vi "Lab Panel V5.28.vi"() -> ()   [LabVIEW 2013] (continued)
                          frame False {
                          }
                          frame True {
                            n3233 = Multiply(x=w5908, y=w5907) -> (x*y=w5906:dbl)
                            n3234 = Multiply(x=w5908, y=w5910) -> (x*y=w5909:dbl)
                          }
                        }
                        n3235 = case shown="True" w5876 {
                          tunnel: w5884 -> [w5912 w5917]
                          tunnel: w5885 -> [_ w5915]
                          tunnel: [w5912 w5916] -> w5882
                          tunnel: w5883 -> [w5911 w5914]
                          tunnel: [w5911 w5913] -> w5881
                          frame False {
                          }
                          frame True {
                            n3236 = Multiply(x=w5915, y=w5914) -> (x*y=w5913:dbl)
                            n3237 = Multiply(x=w5915, y=w5917) -> (x*y=w5916:dbl)
                          }
                        }
                        n3238 = local read "SIG LAB03-2"() -> (w5900:T2)
                        n3239 = local read "SIG LAB03-1"() -> (w5902:T2)
                        n3240 = Bundle By Name(cluster=w5902, "Tmp Live"=w5882, "Tmp Neut"=w5881) -> (w5901:T2)
                        n3241 = Bundle By Name(cluster=w5900, "Tmp Live"=w5878, "Tmp Neut"=w5877) -> (w5899:T2)
                        n3242 = local write "SIG LAB03-1"(w5901) -> ()
                        n3243 = local write "SIG LAB03-2"(w5899) -> ()
                      }
                      frame #4 {
                        n3244 = case shown="False" w5932 {
                          tunnel: [w5963 w5964] -> w5948
                          tunnel: w5931 -> [_ w5964]
                          frame False {
                            n3245 = local read "CAL LAB04"() -> (w5963:T14)
                          }
                          frame True {
                          }
                        }
                        n3246 = local read "LAB04 TEMP"() -> (w5938:T12)
                        n3247 = local read "TEMP LA04"() -> (w5939:T9)
                        n3248 = call "sub vi - temperature delay v4.vi"("2-run"=w5920, "1-run"=w5921, "temp values IN"=w5939, "temp signals"=w5938) -> ("T2-N"=w5933:dbl, "T2-L"=w5934:dbl, "T1-N"=w5935:dbl, "T1-L"=w5936:dbl, "temp values OUT"=w5937:T44)  [unwired: 3 in]
                        n3249 = Unbundle By Name(w5948) -> ("1 (TL) cal"=w5943:dbl, "1 (TN) cal"=w5942:dbl, "2 (TL) cal"=w5941:dbl, "2 (TN) cal"=w5940:dbl)  [unwired: 6 out]
                        n3250 = local write "TEMP LA04"(w5937) -> ()
                        n3251 = Multiply(x=w5936, y=w5943) -> (x*y=w5929:dbl)
                        n3252 = Multiply(x=w5935, y=w5942) -> (x*y=w5928:dbl)
                        n3253 = Multiply(x=w5934, y=w5941) -> (x*y=w5925:dbl)
                        n3254 = Multiply(x=w5933, y=w5940) -> (x*y=w5924:dbl)
                        n3255 = case shown="True" w5920 {
                          tunnel: w5925 -> [w5950 w5955]
                          tunnel: w5930 -> [_ w5953]
                          tunnel: [w5950 w5954] -> w5923
                          tunnel: w5924 -> [w5949 w5952]
                          tunnel: [w5949 w5951] -> w5922
                          frame False {
                          }
                          frame True {
                            n3256 = Multiply(x=w5953, y=w5952) -> (x*y=w5951:dbl)
                            n3257 = Multiply(x=w5953, y=w5955) -> (x*y=w5954:dbl)
                          }
                        }
                        n3258 = case shown="True" w5921 {
                          tunnel: w5929 -> [w5957 w5962]
                          tunnel: w5930 -> [_ w5960]
                          tunnel: [w5957 w5961] -> w5927
                          tunnel: w5928 -> [w5956 w5959]
                          tunnel: [w5956 w5958] -> w5926
                          frame False {
                          }
                          frame True {
                            n3259 = Multiply(x=w5960, y=w5959) -> (x*y=w5958:dbl)
                            n3260 = Multiply(x=w5960, y=w5962) -> (x*y=w5961:dbl)
                          }
                        }
                        n3261 = local read "SIG LAB04-2"() -> (w5945:T2)
                        n3262 = local read "SIG LAB04-1"() -> (w5947:T2)
                        n3263 = Bundle By Name(cluster=w5947, "Tmp Live"=w5927, "Tmp Neut"=w5926) -> (w5946:T2)
                        n3264 = Bundle By Name(cluster=w5945, "Tmp Live"=w5923, "Tmp Neut"=w5922) -> (w5944:T2)
                        n3265 = local write "SIG LAB04-1"(w5946) -> ()
                        n3266 = local write "SIG LAB04-2"(w5944) -> ()
                      }
                      frame #5 {
                        n3267 = case shown="False" w5977 {
                          tunnel: [w6008 w6009] -> w5993
                          tunnel: w5976 -> [_ w6009]
                          frame False {
                            n3268 = local read "CAL LAB05"() -> (w6008:T14)
                          }
                          frame True {
                          }
                        }
                        n3269 = local read "LAB05 TEMP"() -> (w5983:T12)
                        n3270 = local read "TEMP LA05"() -> (w5984:T9)
                        n3271 = call "sub vi - temperature delay v4.vi"("2-run"=w5965, "1-run"=w5966, "temp values IN"=w5984, "temp signals"=w5983) -> ("T2-N"=w5979:dbl, "T2-L"=w5980:dbl, "T1-N"=w5981:dbl, "T1-L"=w5982:dbl, "temp values OUT"=w5978:T44)  [unwired: 3 in]
                        n3272 = local write "TEMP LA05"(w5978) -> ()
                        n3273 = Unbundle By Name(w5993) -> ("1 (TL) cal"=w5985:dbl, "1 (TN) cal"=w5988:dbl, "2 (TL) cal"=w5987:dbl, "2 (TN) cal"=w5986:dbl)  [unwired: 6 out]
                        n3274 = Multiply(x=w5982, y=w5985) -> (x*y=w5974:dbl)
                        n3275 = Multiply(x=w5981, y=w5988) -> (x*y=w5973:dbl)
                        n3276 = Multiply(x=w5980, y=w5987) -> (x*y=w5970:dbl)
                        n3277 = Multiply(x=w5979, y=w5986) -> (x*y=w5969:dbl)
                        n3278 = case shown="True" w5965 {
                          tunnel: w5970 -> [w5995 w6000]
                          tunnel: w5975 -> [_ w5998]
                          tunnel: [w5995 w5999] -> w5968
                          tunnel: w5969 -> [w5994 w5997]
                          tunnel: [w5994 w5996] -> w5967
                          frame False {
                          }
                          frame True {
                            n3279 = Multiply(x=w5998, y=w5997) -> (x*y=w5996:dbl)
                            n3280 = Multiply(x=w5998, y=w6000) -> (x*y=w5999:dbl)
                          }
                        }
                        n3281 = case shown="True" w5966 {
                          tunnel: w5974 -> [w6002 w6007]
                          tunnel: w5975 -> [_ w6005]
                          tunnel: [w6002 w6006] -> w5972
                          tunnel: w5973 -> [w6001 w6004]
                          tunnel: [w6001 w6003] -> w5971
                          frame False {
                          }
                          frame True {
                            n3282 = Multiply(x=w6005, y=w6004) -> (x*y=w6003:dbl)
                            n3283 = Multiply(x=w6005, y=w6007) -> (x*y=w6006:dbl)
                          }
                        }
                        n3284 = local read "SIG LAB05-1"() -> (w5992:T2)
                        n3285 = Bundle By Name(cluster=w5992, "Tmp Live"=w5972, "Tmp Neut"=w5971) -> (w5991:T2)
                        n3286 = local read "SIG LAB05-2"() -> (w5990:T2)
                        n3287 = Bundle By Name(cluster=w5990, "Tmp Live"=w5968, "Tmp Neut"=w5967) -> (w5989:T2)
                        n3288 = local write "SIG LAB05-1"(w5991) -> ()
                        n3289 = local write "SIG LAB05-2"(w5989) -> ()
                      }
                      frame #6 {
                        w6110 = 150.0
                        # "check for thermocouple error, output >150 deg??"
                        n3290 = local read "SIG LAB01-2"() -> (w6119:T2)
                        n3291 = local read "SIG LAB04-1"() -> (w6113:T2)
                        n3292 = local read "SIG LAB04-2"() -> (w6114:T2)
                        n3293 = local read "SIG LAB01-1"() -> (w6120:T2)
                        n3294 = Unbundle(w6114) -> ("Tmp Live"=w6024:dbl, "Tmp Neut"=w6023:dbl)  [unwired: 3 out]
                        n3295 = Unbundle(w6119) -> ("Tmp Live"=w6045:dbl, "Tmp Neut"=w6043:dbl)  [unwired: 3 out]
                        n3296 = Unbundle(w6113) -> ("Tmp Live"=w6025:dbl, "Tmp Neut"=w6018:dbl)  [unwired: 3 out]
                        n3297 = Unbundle(w6120) -> ("Tmp Live"=w6048:dbl, "Tmp Neut"=w6046:dbl)  [unwired: 3 out]
                        n3298 = Absolute Value(x=w6025) -> (abs(x)=w6019:dbl)
                        n3299 = Absolute Value(x=w6018) -> (abs(x)=w6020:dbl)
                        n3300 = Absolute Value(x=w6024) -> (abs(x)=w6022:dbl)
                        n3301 = Absolute Value(x=w6023) -> (abs(x)=w6021:dbl)
                        n3302 = Absolute Value(x=w6045) -> (abs(x)=w6044:dbl)
                        n3303 = Absolute Value(x=w6043) -> (abs(x)=w6042:dbl)
                        n3304 = Absolute Value(x=w6046) -> (abs(x)=w6047:dbl)
                        n3305 = Absolute Value(x=w6048) -> (abs(x)=w6049:dbl)
                        n3306 = Greater?(x=w6021, y=w6110) -> (0:w6086:bool)
                        "LA04-2 (TN)" <- w6086
                        n3307 = Greater?(x=w6042, y=w6110) -> (0:w6098:bool)
                        "LA01-2 (TN)" <- w6098
                        n3308 = Greater?(x=w6022, y=w6110) -> (0:w6087:bool)
                        "LA04-2 (TL)" <- w6087
                        n3309 = Greater?(x=w6044, y=w6110) -> (0:w6099:bool)
                        "LA01-2 (TL)" <- w6099
                        n3310 = Greater?(x=w6020, y=w6110) -> (0:w6088:bool)
                        "LA04-1 (TN)" <- w6088
                        n3311 = Greater?(x=w6047, y=w6110) -> (0:w6109:bool)
                        "LA01-1 (TN)" <- w6109
                        n3312 = Greater?(x=w6019, y=w6110) -> (0:w6089:bool)
                        "LA04-1 (TL)" <- w6089
                        n3313 = Greater?(x=w6049, y=w6110) -> (0:w6108:bool)
                        "LA01-1 (TL)" <- w6108
                        n3314 = Or(x=w6109, y=w6108) -> (x .or. y?=w6107:bool)
                        n3315 = Or(x=w6086, y=w6087) -> (x .or. y?=w6097:bool)
                        n3316 = Or(x=w6099, y=w6098) -> (x .or. y?=w6103:bool)
                        n3317 = Or(x=w6088, y=w6089) -> (x .or. y?=w6093:bool)
                        n3318 = Select(t=u32 16711680, s=w6107, f=u32 13816530) -> (s? t:f=w6104:u32)
                        n3319 = Select(t=u32 16711680, s=w6097, f=u32 13816530) -> (s? t:f=w6094:u32)
                        n3320 = Select(t=u32 16711680, s=w6103, f=u32 13816530) -> (s? t:f=w6100:u32)
                        n3321 = Select(t=u32 16711680, s=w6093, f=u32 13816530) -> (s? t:f=w6090:u32)
                        n3322 = property on="SIG LAB01-1" class="Clust (strict)"("Color"=w6104) -> ()  [unwired: 2 in, 2 out]
                        n3323 = property on="SIG LAB01-2" class="Clust (strict)"("Color"=w6100) -> ()  [unwired: 2 in, 2 out]
                        n3324 = property on="SIG LAB04-2" class="Clust (strict)"("Color"=w6094) -> ()  [unwired: 2 in, 2 out]
                        n3325 = property on="SIG LAB04-1" class="Clust (strict)"("Color"=w6090) -> ()  [unwired: 2 in, 2 out]
                        n3326 = local read "SIG LAB02-1"() -> (w6117:T2)
                        n3327 = local read "SIG LAB02-2"() -> (w6118:T2)
                        n3328 = local read "SIG LAB05-2"() -> (w6111:T2)
                        n3329 = local read "SIG LAB05-1"() -> (w6112:T2)
                        n3330 = Unbundle(w6118) -> ("Tmp Live"=w6037:dbl, "Tmp Neut"=w6035:dbl)  [unwired: 3 out]
                        n3331 = Unbundle(w6117) -> ("Tmp Live"=w6041:dbl, "Tmp Neut"=w6040:dbl)  [unwired: 3 out]
                        n3332 = Unbundle(w6111) -> ("Tmp Live"=w6013:dbl, "Tmp Neut"=w6011:dbl)  [unwired: 3 out]
                        n3333 = Unbundle(w6112) -> ("Tmp Live"=w6017:dbl, "Tmp Neut"=w6015:dbl)  [unwired: 3 out]
                        n3334 = Absolute Value(x=w6037) -> (abs(x)=w6036:dbl)
                        n3335 = Absolute Value(x=w6035) -> (abs(x)=w6034:dbl)
                        n3336 = Absolute Value(x=w6040) -> (abs(x)=w6038:dbl)
                        n3337 = Absolute Value(x=w6041) -> (abs(x)=w6039:dbl)
                        n3338 = Absolute Value(x=w6013) -> (abs(x)=w6012:dbl)
                        n3339 = Absolute Value(x=w6011) -> (abs(x)=w6010:dbl)
                        n3340 = Absolute Value(x=w6017) -> (abs(x)=w6016:dbl)
                        n3341 = Absolute Value(x=w6015) -> (abs(x)=w6014:dbl)
                        n3342 = Greater?(x=w6034, y=w6110) -> (0:w6062:bool)
                        "LA02-2 (TN)" <- w6062
                        n3343 = Greater?(x=w6036, y=w6110) -> (0:w6063:bool)
                        "LA02-2 (TL)" <- w6063
                        n3344 = Greater?(x=w6038, y=w6110) -> (0:w6065:bool)
                        "LA02-1 (TN)" <- w6065
                        n3345 = Greater?(x=w6039, y=w6110) -> (0:w6064:bool)
                        "LA02-1 (TL)" <- w6064
                        n3346 = Greater?(x=w6010, y=w6110) -> (0:w6074:bool)
                        "LA05-2 (TN)" <- w6074
                        n3347 = Greater?(x=w6012, y=w6110) -> (0:w6075:bool)
                        "LA05-2 (TL)" <- w6075
                        n3348 = Greater?(x=w6014, y=w6110) -> (0:w6076:bool)
                        "LA05-1 (TN)" <- w6076
                        n3349 = Greater?(x=w6016, y=w6110) -> (0:w6077:bool)
                        "LA05-1 (TL)" <- w6077
                        n3350 = Or(x=w6065, y=w6064) -> (x .or. y?=w6073:bool)
                        n3351 = Or(x=w6063, y=w6062) -> (x .or. y?=w6069:bool)
                        n3352 = Or(x=w6077, y=w6076) -> (x .or. y?=w6085:bool)
                        n3353 = Or(x=w6075, y=w6074) -> (x .or. y?=w6081:bool)
                        n3354 = Select(t=u32 16711680, s=w6073, f=u32 13816530) -> (s? t:f=w6070:u32)
                        n3355 = Select(t=u32 16711680, s=w6069, f=u32 13816530) -> (s? t:f=w6066:u32)
                        n3356 = Select(t=u32 16711680, s=w6085, f=u32 13816530) -> (s? t:f=w6082:u32)
                        n3357 = Select(t=u32 16711680, s=w6081, f=u32 13816530) -> (s? t:f=w6078:u32)
                        n3358 = local read "SIG LAB03-1"() -> (w6115:T2)
                        n3359 = property on="SIG LAB02-1" class="Clust (strict)"("Color"=w6070) -> ()  [unwired: 2 in, 2 out]
                        n3360 = property on="SIG LAB02-2" class="Clust (strict)"("Color"=w6066) -> ()  [unwired: 2 in, 2 out]
                        n3361 = local read "SIG LAB03-2"() -> (w6116:T2)
                        n3362 = property on="SIG LAB05-1" class="Clust (strict)"("Color"=w6082) -> ()  [unwired: 2 in, 2 out]
                        n3363 = property on="SIG LAB05-2" class="Clust (strict)"("Color"=w6078) -> ()  [unwired: 2 in, 2 out]
                        n3364 = Unbundle(w6116) -> ("Tmp Live"=w6029:dbl, "Tmp Neut"=w6027:dbl)  [unwired: 3 out]
                        n3365 = Unbundle(w6115) -> ("Tmp Live"=w6033:dbl, "Tmp Neut"=w6031:dbl)  [unwired: 3 out]
                        n3366 = Absolute Value(x=w6029) -> (abs(x)=w6028:dbl)
                        n3367 = Absolute Value(x=w6027) -> (abs(x)=w6026:dbl)
                        n3368 = Absolute Value(x=w6033) -> (abs(x)=w6032:dbl)
                        n3369 = Absolute Value(x=w6031) -> (abs(x)=w6030:dbl)
                        n3370 = Greater?(x=w6026, y=w6110) -> (0:w6050:bool)
                        "LA03-2 (TN)" <- w6050
                        n3371 = Greater?(x=w6028, y=w6110) -> (0:w6051:bool)
                        "LA03-2 (TL)" <- w6051
                        n3372 = Greater?(x=w6030, y=w6110) -> (0:w6053:bool)
                        "LA03-1 (TN)" <- w6053
                        n3373 = Greater?(x=w6032, y=w6110) -> (0:w6052:bool)
                        "LA03-1 (TL)" <- w6052
                        n3374 = Or(x=w6053, y=w6052) -> (x .or. y?=w6061:bool)
                        n3375 = Or(x=w6051, y=w6050) -> (x .or. y?=w6057:bool)
                        n3376 = Select(t=u32 16711680, s=w6061, f=u32 13816530) -> (s? t:f=w6058:u32)
                        n3377 = Select(t=u32 16711680, s=w6057, f=u32 13816530) -> (s? t:f=w6054:u32)
                        n3378 = property on="SIG LAB03-1" class="Clust (strict)"("Color"=w6058) -> ()  [unwired: 2 in, 2 out]
                        n3379 = property on="SIG LAB03-2" class="Clust (strict)"("Color"=w6054) -> ()  [unwired: 2 in, 2 out]
                      }
                    }
                  }
                }
              }
            }
          }
          frame #22 {
            # "SAVE ON AMPS VALUES FOR REPORT FILE"
            # "write data to display panel"
            n3380 = global write "Global display 1.vi" "TEST 5-2"(w6156) -> ()
            n3381 = global write "Global display 1.vi" "TEST 4-2"(w6158) -> ()
            n3382 = global write "Global display 1.vi" "TEST 1-2"(w6164) -> ()
            n3383 = global write "Global display 1.vi" "TEST 3-1"(w6161) -> ()
            n3384 = global write "Global display 1.vi" "TEST 5-1"(w6157) -> ()
            n3385 = global write "Global display 1.vi" "TEST 1-1"(w6165) -> ()
            n3386 = global write "Global display 1.vi" "TEST 3-2"(w6160) -> ()
            n3387 = global write "Global display 1.vi" "TEST 4-1"(w6159) -> ()
            n3388 = global write "Global display 1.vi" "TEST 2-2"(w6162) -> ()
            n3389 = global write "Global display 1.vi" "TEST 2-1"(w6163) -> ()
            n3390 = global read "Global display 3.vi" "log 1-1"() -> (→"LOG LAB01-1":string)
            n3391 = global read "Global display 3.vi" "log 3-1"() -> (→"LOG LAB03-1":string)
            n3392 = global read "Global display 3.vi" "log 1-2"() -> (→"LOG LAB01-2":string)
            n3393 = property on="Tab Control 2" class="TabCtl (strict)"() -> ("Pages"=w6155:refnum<vi>[])  [unwired: 2 in, 2 out]
            n3394 = global read "Global display 3.vi" "log 2-1"() -> (→"LOG LAB02-1":string)
            n3395 = global read "Global display 3.vi" "log 2-2"() -> (→"LOG LAB02-2":string)
            n3396 = global read "Global display 3.vi" "log 4-2"() -> (→"LOG LAB04-2":string)
            n3397 = global read "Global display 3.vi" "log 5-2"() -> (→"LOG LAB05-2":string)
            n3398 = global read "Global display 3.vi" "log 5-1"() -> (→"LOG LAB05-1":string)
            n3399 = global read "Global display 3.vi" "log 4-1"() -> (→"LOG LAB04-1":string)
            n3400 = global read "Global display 3.vi" "log 3-2"() -> (→"LOG LAB03-2":string)
            n3401 = Index Array(array=w6155, index=8) -> (element=w6153:refnum<vi>)
            n3402 = property class="Page"(reference=w6153) -> ("PageVis"=w6152:bool)  [unwired: 1 in, 2 out]
            n3403 = global write "Global display 3.vi" "admin"(w6152) -> ()
            n3404 = local read "O/I  LAB05-2"() -> (w6206:bool)
            n3405 = local read "O/I  LAB05-1"() -> (w6207:bool)
            n3406 = local read "O/I  LAB03-2"() -> (w6210:bool)
            n3407 = local read "O/I  LAB04-2"() -> (w6208:bool)
            n3408 = local read "O/I  LAB04-1"() -> (w6209:bool)
            n3409 = local read "O/I  LAB03-1"() -> (w6211:bool)
            n3410 = local read "O/I  LAB01-2"() -> (w6214:bool)
            n3411 = local read "O/I  LAB01-1"() -> (w6215:bool)
            n3412 = local read "O/I  LAB02-1"() -> (w6213:bool)
            n3413 = local read "O/I  LAB02-2"() -> (w6212:bool)
            n3414 = global write "Global display 1.vi" "5-2 O/F"(w6206) -> ()
            n3415 = global write "Global display 1.vi" "5-1 O/F"(w6207) -> ()
            n3416 = global write "Global display 1.vi" "4-1 O/F"(w6209) -> ()
            n3417 = global write "Global display 1.vi" "4-2 O/F"(w6208) -> ()
            n3418 = global write "Global display 1.vi" "3-2 O/F"(w6210) -> ()
            n3419 = global write "Global display 1.vi" "3-1 O/F"(w6211) -> ()
            n3420 = global write "Global display 1.vi" "2-2 O/F"(w6212) -> ()
            n3421 = global write "Global display 1.vi" "2-1 O/F"(w6213) -> ()
            n3422 = global write "Global display 1.vi" "1-2 O/F"(w6214) -> ()
            n3423 = global write "Global display 1.vi" "1-1 O/F"(w6215) -> ()
            n3424 = local read "TEMP START LAB02-2"() -> (w6138:cluster{"TL":dbl, "TN":dbl})
            n3425 = local read "run lab05-2"() -> (w6196:bool)
            n3426 = local read "TEMP START LAB01-2"() -> (w6140:cluster{"TL":dbl, "TN":dbl})
            n3427 = local read "TEMP START LAB02-1"() -> (w6139:cluster{"TL":dbl, "TN":dbl})
            n3428 = local read "TEMP START LAB04-1"() -> (w6135:cluster{"TL":dbl, "TN":dbl})
            n3429 = local read "TEMP START LAB04-2"() -> (w6134:cluster{"TL":dbl, "TN":dbl})
            n3430 = local read "run lab04-1"() -> (w6199:bool)
            n3431 = local read "run lab04-2"() -> (w6198:bool)
            n3432 = local read "run lab05-1"() -> (w6197:bool)
            n3433 = local read "TEMP START LAB01-1"() -> (w6141:cluster{"TL":dbl, "TN":dbl})
            n3434 = local read "TEMP START LAB05-2"() -> (w6132:cluster{"TL":dbl, "TN":dbl})
            n3435 = local read "TEMP START LAB05-1"() -> (w6133:cluster{"TL":dbl, "TN":dbl})
            n3436 = local read "run lab03-2"() -> (w6200:bool)
            n3437 = local read "TEMP START LAB03-2"() -> (w6136:cluster{"TL":dbl, "TN":dbl})
            n3438 = local read "TEMP START LAB03-1"() -> (w6137:cluster{"TL":dbl, "TN":dbl})
            n3439 = local read "run lab02-1"() -> (w6203:bool)
            n3440 = local read "run lab03-1"() -> (w6201:bool)
            n3441 = local read "run lab01-2"() -> (w6204:bool)
            n3442 = local read "run lab02-2"() -> (w6202:bool)
            n3443 = local read "run lab01-1"() -> (w6205:bool)
            n3444 = global write "Global display 1.vi" "5-2 R/S"(w6196) -> ()
            n3445 = global write "Global display 1.vi" "5-1 R/S"(w6197) -> ()
            n3446 = global write "Global display 1.vi" "4-2 R/S"(w6198) -> ()
            n3447 = global write "Global display 1.vi" "4-1 R/S"(w6199) -> ()
            n3448 = global write "Global display 1.vi" "3-2 R/S"(w6200) -> ()
            n3449 = global write "Global display 1.vi" "1-2 R/S"(w6204) -> ()
            n3450 = global write "Global display 1.vi" "2-1 R/S"(w6203) -> ()
            n3451 = global write "Global display 1.vi" "3-1 R/S"(w6201) -> ()
            n3452 = global write "Global display 1.vi" "2-2 R/S"(w6202) -> ()
            n3453 = global write "Global display 1.vi" "1-1 R/S"(w6205) -> ()
            n3454 = global write "Global display 3.vi" "TEMP ST 05-2"(w6132) -> ()
            n3455 = global write "Global display 3.vi" "TEMP ST 05-1"(w6133) -> ()
            n3456 = global write "Global display 3.vi" "TEMP ST 03-2"(w6136) -> ()
            n3457 = global write "Global display 3.vi" "TEMP ST 04-2"(w6134) -> ()
            n3458 = global write "Global display 3.vi" "TEMP ST 01-1"(w6141) -> ()
            n3459 = global write "Global display 3.vi" "TEMP ST 01-2"(w6140) -> ()
            n3460 = global write "Global display 3.vi" "TEMP ST 04-1"(w6135) -> ()
            n3461 = global write "Global display 3.vi" "TEMP ST 02-1"(w6139) -> ()
            n3462 = global write "Global display 3.vi" "TEMP ST 02-2"(w6138) -> ()
            n3463 = global write "Global display 3.vi" "TEMP ST 03-1"(w6137) -> ()
            n3464 = local read "DISP LAB04-2"() -> (w6188:T4)
            n3465 = local read "DISP LAB05-1"() -> (w6187:T4)
            n3466 = local read "DISP LAB04-1"() -> (w6189:T4)
            n3467 = local read "DISP LAB05-2"() -> (w6186:T4)
            n3468 = local read "DISP LAB03-2"() -> (w6190:T4)
            n3469 = local read "DISP LAB03-1"() -> (w6191:T4)
            n3470 = local read "DISP LAB01-2"() -> (w6194:T4)
            n3471 = local read "DISP LAB02-1"() -> (w6193:T4)
            n3472 = local read "DISP LAB02-2"() -> (w6192:T4)
            n3473 = local read "DISP LAB01-1"() -> (w6195:T4)
            n3474 = local read "TEMP RISE LAB05-1"() -> (w6123:cluster{"TL":dbl, "TN":dbl})
            n3475 = local read "TEMP RISE LAB05-2"() -> (w6122:cluster{"TL":dbl, "TN":dbl})
            n3476 = local read "TEMP RISE LAB04-2"() -> (w6124:cluster{"TL":dbl, "TN":dbl})
            n3477 = local read "TEMP RISE LAB04-1"() -> (w6125:cluster{"TL":dbl, "TN":dbl})
            n3478 = local read "TEMP RISE LAB03-2"() -> (w6126:cluster{"TL":dbl, "TN":dbl})
            n3479 = local read "TEMP RISE LAB03-1"() -> (w6127:cluster{"TL":dbl, "TN":dbl})
            n3480 = local read "TEMP RISE LAB01-2"() -> (w6130:cluster{"TL":dbl, "TN":dbl})
            n3481 = local read "TEMP RISE LAB02-2"() -> (w6128:cluster{"TL":dbl, "TN":dbl})
            n3482 = local read "TEMP RISE LAB01-1"() -> (w6131:cluster{"TL":dbl, "TN":dbl})
            n3483 = local read "TEMP RISE LAB02-1"() -> (w6129:cluster{"TL":dbl, "TN":dbl})
            n3484 = global write "Global display 2.vi" "DISP LAB05-1"(w6187) -> ()
            n3485 = global write "Global display 2.vi" "DISP LAB05-2"(w6186) -> ()
            n3486 = global write "Global display 2.vi" "DISP LAB04-2"(w6188) -> ()
            n3487 = global write "Global display 2.vi" "DISP LAB04-1"(w6189) -> ()
            n3488 = global write "Global display 2.vi" "DISP LAB02-1"(w6193) -> ()
            n3489 = global write "Global display 2.vi" "DISP LAB02-2"(w6192) -> ()
            n3490 = global write "Global display 2.vi" "DISP LAB03-2"(w6190) -> ()
            n3491 = global write "Global display 2.vi" "DISP LAB01-2"(w6194) -> ()
            n3492 = global write "Global display 2.vi" "DISP LAB01-1"(w6195) -> ()
            n3493 = global write "Global display 2.vi" "DISP LAB03-1"(w6191) -> ()
            n3494 = global write "Global display 3.vi" "TEMP RS 05-2"(w6122) -> ()
            n3495 = global write "Global display 3.vi" "TEMP RS 05-1"(w6123) -> ()
            n3496 = global write "Global display 3.vi" "TEMP RS 03-2"(w6126) -> ()
            n3497 = global write "Global display 3.vi" "TEMP RS 02-1"(w6129) -> ()
            n3498 = global write "Global display 3.vi" "TEMP RS 02-2"(w6128) -> ()
            n3499 = global write "Global display 3.vi" "TEMP RS 04-2"(w6124) -> ()
            n3500 = global write "Global display 3.vi" "TEMP RS 01-2"(w6130) -> ()
            n3501 = global write "Global display 3.vi" "TEMP RS 03-1"(w6127) -> ()
            n3502 = global write "Global display 3.vi" "TEMP RS 04-1"(w6125) -> ()
            n3503 = global write "Global display 3.vi" "TEMP RS 01-1"(w6131) -> ()
            n3504 = local read "SET LAB05-2"() -> (w6176:T5)
            n3505 = local read "SET LAB05-1"() -> (w6177:T5)
            n3506 = local read "SET LAB04-1"() -> (w6179:T5)
            n3507 = local read "SET LAB04-2"() -> (w6178:T5)
            n3508 = local read "SET LAB01-1"() -> (w6185:T5)
            n3509 = local read "SET LAB03-1"() -> (w6181:T5)
            n3510 = local read "SET LAB03-2"() -> (w6180:T5)
            n3511 = local read "SET LAB02-2"() -> (w6182:T5)
            n3512 = local read "SET LAB01-2"() -> (w6184:T5)
            n3513 = local read "SET LAB02-1"() -> (w6183:T5)
            n3514 = global write "Global display 2.vi" "SET LAB05-2"(w6176) -> ()
            n3515 = global write "Global display 2.vi" "SET LAB05-1"(w6177) -> ()
            n3516 = global write "Global display 2.vi" "SET LAB04-1"(w6179) -> ()
            n3517 = global write "Global display 2.vi" "SET LAB01-1"(w6185) -> ()
            n3518 = global write "Global display 2.vi" "SET LAB04-2"(w6178) -> ()
            n3519 = global write "Global display 2.vi" "SET LAB03-2"(w6180) -> ()
            n3520 = global write "Global display 2.vi" "SET LAB02-2"(w6182) -> ()
            n3521 = global write "Global display 2.vi" "SET LAB03-1"(w6181) -> ()
            n3522 = global write "Global display 2.vi" "SET LAB01-2"(w6184) -> ()
            n3523 = global write "Global display 2.vi" "SET LAB02-1"(w6183) -> ()
            n3524 = local read "RESULT LAB01-1"() -> (w6175:bool)
            n3525 = local read "RESULT LAB03-2"() -> (w6170:bool)
            n3526 = local read "RESULT LAB04-1"() -> (w6169:bool)
            n3527 = local read "RESULT LAB04-2"() -> (w6168:bool)
            n3528 = local read "RESULT LAB02-2"() -> (w6172:bool)
            n3529 = local read "RESULT LAB01-2"() -> (w6174:bool)
            n3530 = local read "RESULT LAB02-1"() -> (w6173:bool)
            n3531 = local read "RESULT LAB03-1"() -> (w6171:bool)
            n3532 = local read "RESULT LAB05-1"() -> (w6167:bool)
            n3533 = local read "RESULT LAB05-2"() -> (w6166:bool)
            n3534 = global write "Global display 2.vi" "RESULT LAB05-1"(w6167) -> ()
            n3535 = global write "Global display 2.vi" "RESULT LAB01-2"(w6174) -> ()
            n3536 = global write "Global display 2.vi" "RESULT LAB03-2"(w6170) -> ()
            n3537 = global write "Global display 2.vi" "RESULT LAB04-1"(w6169) -> ()
            n3538 = global write "Global display 2.vi" "RESULT LAB04-2"(w6168) -> ()
            n3539 = global write "Global display 2.vi" "RESULT LAB05-2"(w6166) -> ()
            n3540 = global write "Global display 2.vi" "RESULT LAB03-1"(w6171) -> ()
            n3541 = global write "Global display 2.vi" "RESULT LAB02-1"(w6173) -> ()
            n3542 = global write "Global display 2.vi" "RESULT LAB02-2"(w6172) -> ()
            n3543 = global write "Global display 2.vi" "RESULT LAB01-1"(w6175) -> ()
            n3544 = local read "Amps Fail level"() -> (w6121:dbl)
            n3545 = stacked-sequence {
              tunnel: w6121 -> [w6217 w6222 w6227 w6232 w6237 w6242 w6247 w6252 w6257 w6262]
              frame #0 {
                n3546 = local read "SIG LAB01-1"() -> (w6219:T2)
                n3547 = Unbundle(w6219) -> ("AMPS"=w6218:dbl)  [unwired: 4 out]
                n3548 = Greater?(x=w6218, y=w6217) -> (0:w6216:bool)
                n3549 = case shown="True" w6216 {
                  frame False {
                  }
                  frame True {
                    n3550 = local read "ON L01-1"() -> (w6220:cluster{"amps":dbl, "volts":dbl, "pf":dbl})
                    n3551 = global write "Global display 2.vi" "ON L01-1"(w6220) -> ()
                  }
                }
              }
              frame #1 {
                n3552 = local read "SIG LAB01-2"() -> (w6224:T2)
                n3553 = Unbundle(w6224) -> ("AMPS"=w6223:dbl)  [unwired: 4 out]
                n3554 = Greater?(x=w6223, y=w6222) -> (0:w6221:bool)
                n3555 = case shown="True" w6221 {
                  frame False {
                  }
                  frame True {
                    n3556 = local read "ON L01-2"() -> (w6225:cluster{"amps":dbl, "volts":dbl, "pf":dbl})
                    n3557 = global write "Global display 2.vi" "ON L01-2"(w6225) -> ()
                  }
                }
              }
              frame #2 {
                n3558 = local read "SIG LAB02-1"() -> (w6229:T2)
                n3559 = Unbundle(w6229) -> ("AMPS"=w6228:dbl)  [unwired: 4 out]
                n3560 = Greater?(x=w6228, y=w6227) -> (0:w6226:bool)
                n3561 = case shown="True" w6226 {
                  frame False {
                  }
                  frame True {
                    n3562 = local read "ON L02-1"() -> (w6230:cluster{"amps":dbl, "volts":dbl, "pf":dbl})
                    n3563 = global write "Global display 2.vi" "ON L02-1"(w6230) -> ()
                  }
                }
              }
              frame #3 {
                n3564 = local read "SIG LAB02-2"() -> (w6234:T2)
                n3565 = Unbundle(w6234) -> ("AMPS"=w6233:dbl)  [unwired: 4 out]
                n3566 = Greater?(x=w6233, y=w6232) -> (0:w6231:bool)
                n3567 = case shown="True" w6231 {
                  frame False {
                  }
                  frame True {
                    n3568 = local read "ON L02-2"() -> (w6235:cluster{"amps":dbl, "volts":dbl, "pf":dbl})
                    n3569 = global write "Global display 2.vi" "ON L02-2"(w6235) -> ()
                  }
                }
              }
              frame #4 {
                n3570 = local read "SIG LAB03-1"() -> (w6239:T2)
                n3571 = Unbundle(w6239) -> ("AMPS"=w6238:dbl)  [unwired: 4 out]
                n3572 = Greater?(x=w6238, y=w6237) -> (0:w6236:bool)
                n3573 = case shown="True" w6236 {
                  frame False {
                  }
                  frame True {
                    n3574 = local read "ON L03-1"() -> (w6240:cluster{"amps":dbl, "volts":dbl, "pf":dbl})
                    n3575 = global write "Global display 2.vi" "ON L03-1"(w6240) -> ()
                  }
                }
              }
              frame #5 {
                n3576 = local read "SIG LAB03-2"() -> (w6244:T2)
                n3577 = Unbundle(w6244) -> ("AMPS"=w6243:dbl)  [unwired: 4 out]
                n3578 = Greater?(x=w6243, y=w6242) -> (0:w6241:bool)
                n3579 = case shown="True" w6241 {
                  frame False {
                  }
                  frame True {
                    n3580 = local read "ON L03-2"() -> (w6245:cluster{"amps":dbl, "volts":dbl, "pf":dbl})
                    n3581 = global write "Global display 2.vi" "ON L03-2"(w6245) -> ()
                  }
                }
              }
              frame #6 {
                n3582 = local read "SIG LAB04-1"() -> (w6249:T2)
                n3583 = Unbundle(w6249) -> ("AMPS"=w6248:dbl)  [unwired: 4 out]
                n3584 = Greater?(x=w6248, y=w6247) -> (0:w6246:bool)
                n3585 = case shown="True" w6246 {
                  frame False {
                  }
                  frame True {
                    n3586 = local read "ON L04-1"() -> (w6250:cluster{"amps":dbl, "volts":dbl, "pf":dbl})
                    n3587 = global write "Global display 2.vi" "ON L04-1"(w6250) -> ()
                  }
                }
              }
              frame #7 {
                n3588 = local read "SIG LAB04-2"() -> (w6254:T2)
                n3589 = Unbundle(w6254) -> ("AMPS"=w6253:dbl)  [unwired: 4 out]
                n3590 = Greater?(x=w6253, y=w6252) -> (0:w6251:bool)
                n3591 = case shown="True" w6251 {
                  frame False {
                  }
                  frame True {
                    n3592 = local read "ON L04-2"() -> (w6255:cluster{"amps":dbl, "volts":dbl, "pf":dbl})
                    n3593 = global write "Global display 2.vi" "ON L04-2"(w6255) -> ()
                  }
                }
              }
              frame #8 {
                n3594 = local read "SIG LAB05-1"() -> (w6259:T2)
                n3595 = Unbundle(w6259) -> ("AMPS"=w6258:dbl)  [unwired: 4 out]
                n3596 = Greater?(x=w6258, y=w6257) -> (0:w6256:bool)
                n3597 = case shown="True" w6256 {
                  frame False {
                  }
                  frame True {
                    n3598 = local read "ON L05-1"() -> (w6260:cluster{"amps":dbl, "volts":dbl, "pf":dbl})
                    n3599 = global write "Global display 2.vi" "ON L05-1"(w6260) -> ()
                  }
                }
              }
              frame #9 {
                n3600 = local read "SIG LAB05-2"() -> (w6264:T2)
                n3601 = Unbundle(w6264) -> ("AMPS"=w6263:dbl)  [unwired: 4 out]
                n3602 = Greater?(x=w6263, y=w6262) -> (0:w6261:bool)
                n3603 = case shown="True" w6261 {
                  frame False {
                  }
                  frame True {
                    n3604 = local read "ON L05-2"() -> (w6265:cluster{"amps":dbl, "volts":dbl, "pf":dbl})
                    n3605 = global write "Global display 2.vi" "ON L05-2"(w6265) -> ()
                  }
                }
              }
            }
          }
          frame #23 {
            # "simulate values"
            n3606 = global write "Global display 4.vi" "LAB deg C"("LAB deg C") -> ()
          }
          frame #24 {
            # "end main and display program"
            n3607 = stacked-sequence {
              seq-local: [_ w6272 _] -> [_ _ w6278]
              tunnel: w6268 -> [w6269 _ _]
              tunnel: w6267 -> [_ _ w6276]
              frame #0 {
                n3608 = case shown="True" w6269 {
                  frame False {
                  }
                  frame True {
                    n3609 = One Button Dialog(message="Excessive number of USB \nresets done, re-start program.") -> ()  [unwired: 1 in, 1 out]
                  }
                }
              }
              frame #1 {
                # "check for reset error"
                n3610 = local read "Simulate"() -> (w6271:bool)
                n3611 = case shown="False" w6271 {
                  tunnel: [w6273 FALSE] -> w6272
                  frame False {
                    n3612 = local read "Reset Error"() -> (w6273:bool)
                    n3613 = case shown="True" w6273 {
                      frame False {
                      }
                      frame True {
                        n3614 = One Button Dialog(message="USB ERROR, program will be stopped.\nClose program, close windows, switch panel off\nand re power panel. If error persists seek help.") -> ()  [unwired: 1 in, 1 out]
                      }
                    }
                  }
                  frame True {
                  }
                }
              }
              frame #2 {
                # "end labview session"
                n3615 = case shown="True" w6276 {
                  frame False {
                  }
                  frame True {
                    n3616 = call "sub vi - AI USB4704 (3)  Close Task v2.vi"() -> ()  [unwired: 16 in]
                  }
                }
                n3617 = Or(x=w6278, y="stop all") -> (x .or. y?=w6277:bool)
                n3618 = case shown="True" w6277 {
                  frame False {
                  }
                  frame True {
                    n3619 = stacked-sequence {
                      frame #0 {
                        n3620 = global write "Global display 1.vi" "stop disp"(TRUE) -> ()
                      }
                      frame #1 {
                        n3621 = call "sub vi - AI USB4704 (3)  Close Task v2.vi"() -> ()  [unwired: 16 in]
                      }
                      frame #2 {
                        n3622 = Quit LabVIEW(quit? (T)=TRUE) -> ()
                      }
                    }
                  }
                }
              }
            }
          }
        }
        n3623 = node-c288() -> ()  [unwired: 1 in, 1 out]
        "loops" <- w346
      }
      n3624 = node-c288(w318) -> ()  [unwired: 1 out]
    }
  }
